vi "Row Name 2 Write.vi"(4 "error in (no error)":errorcluster, 5 "Value":string, 6 "Container State":T2, 7 "Display State In":T1) -> (0 "error out":errorcluster, 3 "Display State Out":T1)   [LabVIEW 2021, in "roboRIO 10 Bank.xctl"]
uses:
  <vilib>/myRIO/Common/Instrument Driver Framework/Utilities/xctls/roboRIO 10 Bank/roboRIO 10 Bank.xctl
  <vilib>/_xctls/Container State.ctl
  <vilib>/myRIO/Common/Instrument Driver Framework/Utilities/xctls/roboRIO 10 Bank/State.ctl
  <vilib>/_xctls/XControlSupport.lvlib
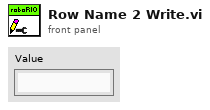
[diagram p1: front panel]
types:
  T1 = typedef "roboRIO 10 Bank.xctl/State.ctl" = cluster{"Pin Disabled?":enum8{"Enabled", "Disabled", "Disabled and Grayed Out"}[], "Pin Name":string[], "Pin ID":string[], "Connector Name":string, "Row Name 1":string, "Row Name 2":string}
  T2 = typedef "XControlSupport.lvlib/Container State.ctl" = cluster{"Indicator?":bool, "Run Mode?":bool, " Refnum":refnum<vi>}
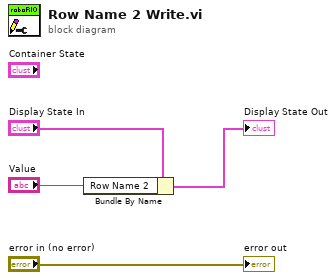
[diagram p0: block diagram]
diagram:
  n1 = Bundle By Name(cluster="Display State In", "Row Name 2"="Value") -> (→"Display State Out":T1)
  "error out" <- "error in (no error)"
